vi "ZLIB Common Path to Specific Path.vi"(10 "common path":string) -> (2 "specific path":path)   [LabVIEW 2019]
panel:
  out "error out":errorcluster
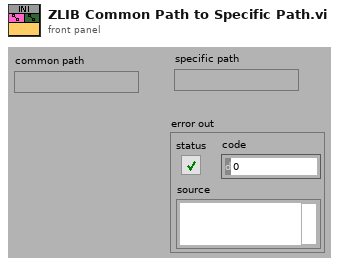
[diagram p1: front panel]
types:
  T1 = enum32{"invalid OS target", "Mac OS", "Windows 3.1", "Windows 95/NT", "Solaris 1", "Solaris 2", "HP-UX", "PowerMAX", "Linux", "Irix", "Rhapsody", "BeOS", "AIX", "OSF1", "VxWorks", "PharLap", "Carbon", "RTX", "Windows x64", "Linux x64", "Mac OS X x64"}
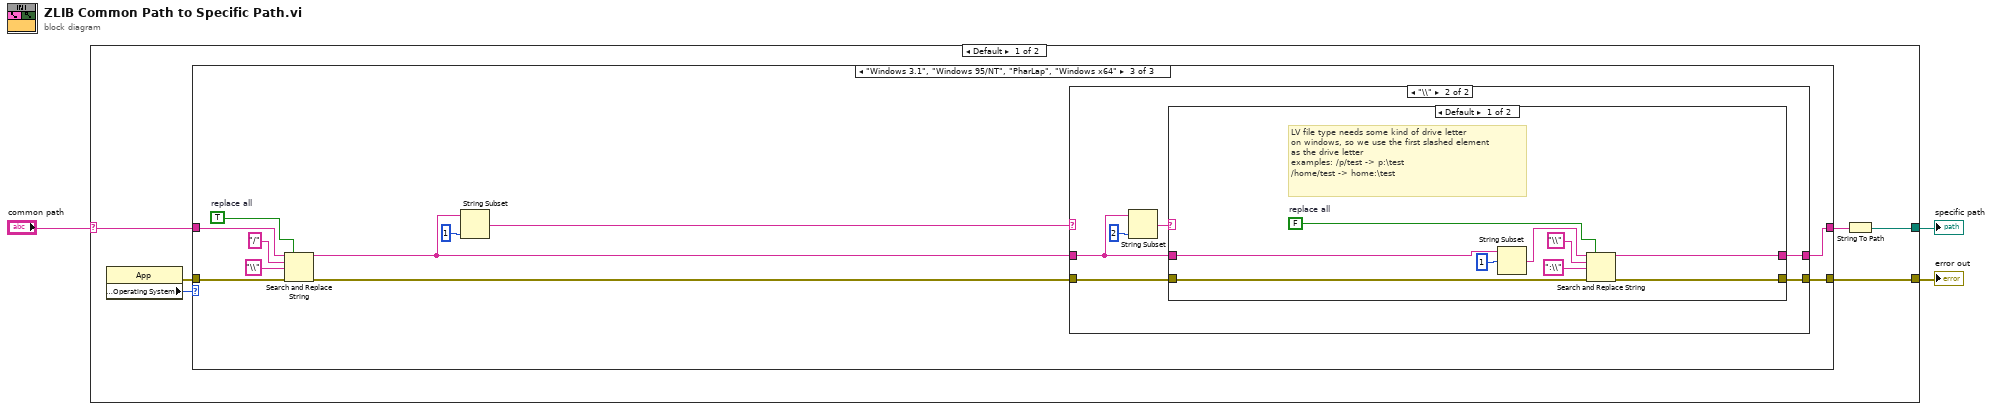
[diagram p0: block diagram]
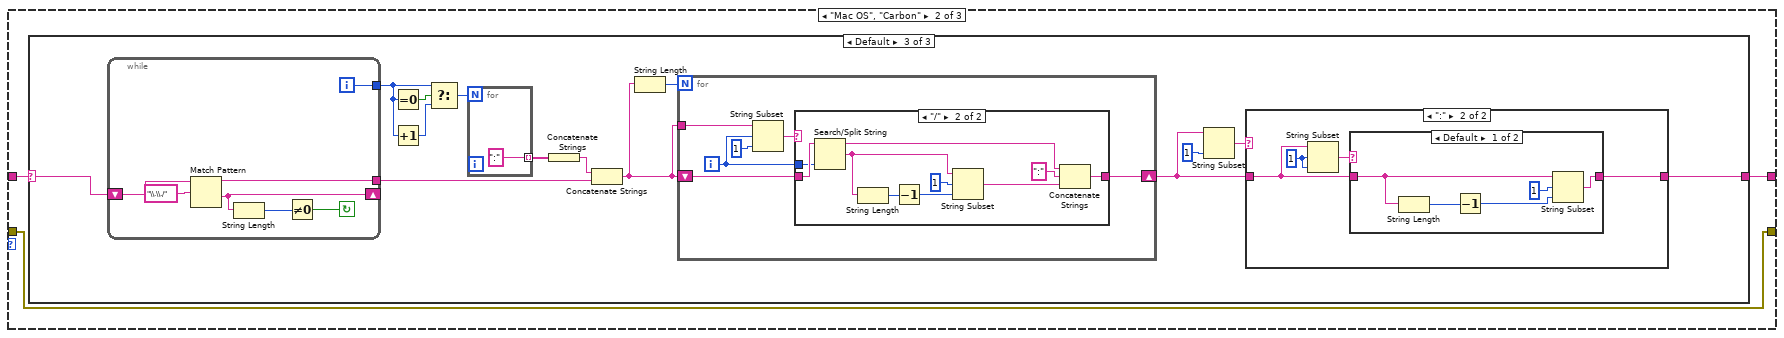
[diagram p3: hidden frame]
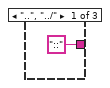
[diagram p4: hidden frame]
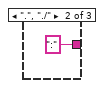
[diagram p5: hidden frame]
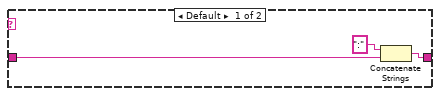
[diagram p7: hidden frame]
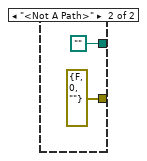
[diagram p11: hidden frame]
diagram:
  n1 = case shown="Default" "common path" {
    selector: "common path" -> [w9 _]
    tunnel: [w8 path "" ("Not A Path Constant")] -> w2
    tunnel: [w4 errorcluster {"status"=FALSE, "code"=0, "source"=""} ("error out")] -> w1
    frame Default {
      n2 = property class="App"() -> (error out=w5:errorcluster, "Application:Target:Operating System"=w6:T1)  [unwired: 2 in, 1 out]
      n3 = case shown="\"Windows 3.1\", \"Windows 95/NT\", \"PharLap\", \"Windows x64\"" w6 {
        tunnel: w9 -> [w11 w14 w76]
        tunnel: [w11 w13 w78] -> w7
        tunnel: w5 -> [w10 w12 w73]
        tunnel: [w10 w12 w69] -> w4
        frame "Linux", "VxWorks", "Linux x64", Default {
        }
        frame "Mac OS", "Carbon" {
          n4 = case shown="Default" w14 {
            selector: w14 -> [_ _ w20]
            tunnel: ["::" ":" w19] -> w13
            frame "..", "../" {
            }
            frame ".", "./" {
            }
            frame Default {
              n5 = while {
                tunnel: [w31] -> w28
                tunnel: [w33] -> w24
                shift-left: w20 -> [w36]
                shift-right: [w32] -> _
                i -> [w31]
                stop <- w34 continue-if-true
                n6 = Match Pattern(string=w36, regular expression="\\.\\./") -> (before substring=w33:string, after substring=w32:string)  [unwired: 3 out]
                n7 = String Length(string=w32) -> (length=w35:i32)
                n8 = Not Equal To 0?(x=w35) -> (x != 0?=w34:bool)
              }
              n9 = Equal To 0?(x=w28) -> (x = 0?=w29:bool)
              n10 = Increment(x=w28) -> (x+1=w27:i32)
              n11 = Select(t=w28, s=w29, f=w27) -> (s? t:f=w26:i32)
              n12 = for {
                N: w26 -> [_]
                tunnel: [":"] -> w25 mode=indexing
              }
              n13 = Concatenate Strings(w25) -> (w18:string)
              n14 = Concatenate Strings(w18, w24) -> (w22:string)
              n15 = String Length(string=w22) -> (length=w23:i32)
              n16 = for {
                N: w23 -> [_]
                tunnel: w22 -> [w41]
                shift-right: [w42] -> w17
                shift-left: w22 -> [w43]
                i -> [w40]
                n17 = String Subset(string=w41, offset (0)=w40, length (rest)=1 ("length")) -> (substring=w38:string)
                n18 = case shown="\"/\"" w38 {
                  tunnel: w43 -> [w44 w54]
                  tunnel: w40 -> [_ w47]
                  tunnel: [w44 w52] -> w42
                  frame Default {
                  }
                  frame "/" {
                    n19 = Search/Split String(string=w54, offset (0)=w47) -> (substring before match=w53:string, match + rest of string=w46:string)  [unwired: 2 out]
                    n20 = String Length(string=w46) -> (length=w50:i32)
                    n21 = Decrement(x=w50) -> (x-1=w49:i32)
                    n22 = String Subset(string=w46, offset (0)=1, length (rest)=w49) -> (substring=w45:string)
                    n23 = Concatenate Strings(w53, ":" ("x"), w45) -> (w52:string)
                  }
                }
              }
              n24 = String Subset(string=w17, length (rest)=1 ("length")) -> (substring=w21:string)  [unwired: 1 out]
              n25 = case shown="\":\"" w21 {
                tunnel: w17 -> [w58 w61]
                tunnel: [w57 w62] -> w19
                frame Default {
                  n26 = Concatenate Strings(":", w58) -> (w57:string)
                }
                frame ":" {
                  w60 = 1 ("length")
                  n27 = String Subset(string=w61, offset (0)=w60, length (rest)=w60) -> (substring=w59:string)
                  n28 = case shown="Default" w59 {
                    tunnel: w61 -> [w63 w68]
                    tunnel: [w64 w68] -> w62
                    frame Default {
                      n29 = String Length(string=w63) -> (length=w66:i32)
                      n30 = Decrement(x=w66) -> (x-1=w65:i32)
                      n31 = String Subset(string=w63, offset (0)=1, length (rest)=w65) -> (substring=w64:string)
                    }
                    frame ":" {
                    }
                  }
                }
              }
            }
          }
        }
        frame "Windows 3.1", "Windows 95/NT", "PharLap", "Windows x64" {
          w72 = TRUE  # replace all
          n32 = Search and Replace String(replace all?=w72, input string=w76, search string="/", replace string="\\" ("replace string (\"\")"), error in=w73) -> (result string=w71:string, error out=w70:errorcluster)  [unwired: 3 in, 2 out]
          n33 = String Subset(string=w71, length (rest)=1 ("length")) -> (substring=w77:string)  [unwired: 1 out]
          n34 = case shown="\"\\\\\"" w77 {
            tunnel: w71 -> [w81 w85]
            tunnel: [w81 w87] -> w78
            tunnel: w70 -> [w80 w83]
            tunnel: [w80 w82] -> w69
            frame Default {
            }
            frame "\\" {
              n35 = String Subset(string=w85, length (rest)=2 ("length")) -> (substring=w84:string)  [unwired: 1 out]
              n36 = case shown="Default" w84 {
                tunnel: w85 -> [w95 w98]
                tunnel: [w96 w98] -> w87
                tunnel: w83 -> [w94 w97]
                tunnel: [w93 w97] -> w82
                frame Default {
                  w90 = FALSE  # replace all
                  # "LV file type needs some kind of drive letter\non windows, so we use the first slashed element\nas the drive letter\nexamples: /p/test -> p:\\test\n/home/test -> home:\\test"
                  n37 = String Subset(string=w95, offset (0)=1) -> (substring=w89:string)  [unwired: 1 in]
                  n38 = Search and Replace String(replace all?=w90, input string=w89, search string="\\", replace string=":\\" ("replace string (\"\")"), error in=w94) -> (result string=w96:string, error out=w93:errorcluster)  [unwired: 3 in, 2 out]
                }
                frame "\\\\" {
                  # "\"\\\\\\\\\" in the case selector corresponds\nto a string value of \\\\"
                }
              }
            }
          }
        }
      }
      n39 = String To Path(string=w7) -> (path=w8:path)
    }
    frame "<Not A Path>" {
    }
  }
  "specific path" <- w2
  "error out" <- w1
